vi "FPGA_Check_Pins_host.vi"() -> ()   [LabVIEW 2018]
uses:
  <vilib>/userdefined/High Color/nirio_resource_hc.ctl
  <vilib>/FPGAPlugInAG/PXI-7951R/niLvFpga_Open_PXI-7951R.vi
  <vilib>/rvi/interface/common/dynamic/niFpgaDynamicAddResources.vi
  <vilib>/FPGAPlugInAG/Dynamic/niLvFpga_Reset_Dynamic.vi
  <vilib>/FPGAPlugInAG/Dynamic/niLvFpga_Run_Dynamic.vi
  <vilib>/Utility/error.llb/Error Cluster From Error Code.vi
  <vilib>/rvi/errors/niLvFpgaAdjustHostInterfaceError.vi
  <vilib>/FPGAPlugInAG/Dynamic/niLvFpga_Close_Dynamic.vi
  <vilib>/rvi/interface/nirviOpenFPGA/nirviOpenFPGA.xnode
  FPGA Bitfiles/FPGACheckPins_FPGATarget_FPGACheckPinstar_hYVdCtpyRbw.lvbitx
  <vilib>/rvi/interface/nirviMethod/nirviMethod.xnode
  <vilib>/rvi/interface/nirviReadWriteControl/nirviReadWriteControl.xnode
  <vilib>/rvi/interface/nirviCloseFPGA/nirviCloseFPGA.xnode
  <vilib>/rvi/interface/Simulation/niFpgaSimulationCallBeginRW.vi
  NiFpgaLv.dll
panel:
  in  "Tab Control":T1(tab)
  out "output array":bool[][](array[boolean])
  out "appended array":bool[](array[boolean])
  out "Ток, А":dbl(knob) scale=0.0..1.0
  in  "FPGA slot name":T2="PXI1Slot2" caption="RIO Device"
  out "error out (4110)":errorcluster
  out "error out FPGA":errorcluster
  in  "Power Resource":refnum<k15>="PXI1Slot3"
  in  "Output enabled CH1":bool
  in  "Stop Program":bool
  in  "Write to Read":bool
  out "Read B":u32=117440511 format="%b"
  out "Read A":u32=134217727 format="%b"
  out "WRITE TOTAL":u32=38686286 format="%b"
  in  "Ток, А  2":dbl=0.9 caption="Current limit CH1" format="%#_13g"
  in  "Напряжение, В":dbl=3.0
  in  "Write to port":u16(ring)=1 items=["Manual mode", "Random", "Increment", "Chess", "NChess", "Only one", "Zero", "Chess diagonal", "NChess diagonal"]
  out "Delay A to B, нс":i16
  out "Delay B to A, нс":i16
  in  "Max тактов":i16
  in  "Write to PFI":u16(ring)=1 items=["Manual mode", "Random", "Increment", "Chess", "NChess", "Only one", "Zero", "Check one"]
  out "Delay 0.0, нс":i16
  out "Delay 0.1, нс":i16
  out "Delay 0.2, нс":i16
  out "Delay 0.3, нс":i16
  out "Delay 0.4, нс":i16
  out "Delay 0.5, нс":i16
  out "Delay 0.6, нс":i16
  out "Delay 0.7, нс":i16
  out "Delay 1.0, нс":i16
  out "Delay 1.1, нс":i16
  out "Delay 1.2, нс":i16
  out "Delay 1.3, нс":i16
  out "Delay 1.4, нс":i16
  out "Delay 1.5, нс":i16
  out "Delay 1.6, нс":i16
  out "Delay 1.7, нс":i16
  out "Delay 2.0, нс":i16
  out "Delay 2.1, нс":i16
  out "Delay 2.2, нс":i16
  out "Delay 2.3, нс":i16
  out "Delay 2.4, нс":i16
  out "Delay 2.5, нс":i16
  out "Delay 2.6, нс":i16
  out "Delay 2.7, нс":i16
  out "Delay PFI1, нс":i16
  out "Delay PFI2, нс":i16
  out "Delay PFI3, нс":i16
  in  "milliseconds to wait":u32
  out "Delay 0.0, нс":i16
  out "Delay 0.1, нс":i16
  out "Delay 0.2, нс":i16
  out "Delay 0.3, нс":i16
  out "Delay 0.4, нс":i16
  out "Delay 0.5, нс":i16
  out "Delay 0.6, нс":i16
  out "Delay 0.7, нс":i16
  out "Delay 1.0, нс":i16
  out "Delay 1.1, нс":i16
  out "Delay 1.2, нс":i16
  out "Delay 1.3, нс":i16
  out "Delay 1.4, нс":i16
  out "Delay 1.5, нс":i16
  out "Delay 1.6, нс":i16
  out "Delay 1.7, нс":i16
  out "Delay 2.0, нс":i16
  out "Delay 2.1, нс":i16
  out "Delay 2.2, нс":i16
  out "Delay 2.3, нс":i16
  out "Delay 2.4, нс":i16
  out "Delay 2.5, нс":i16
  out "Delay 2.6, нс":i16
  out "Delay 2.7, нс":i16
  out "Delay PFI1, нс":i16
  out "Delay PFI2, нс":i16
  out "Delay PFI3, нс":i16
  out "U CH0.1, В":dbl=0.000596728952024882
  out "I CH0.1, A":dbl=2.324707150327661e-06
  in  "Write to PFI 2":u8=6 format="%b"
  in  "Cycle":bool=TRUE
  in  "Write to port  2":u8=248 format="%b"
  out "Read PFI 2":i16=1
  out "Read PFI 3":i16=1
  out "Read PFI 1":i16
  out "Чтение PFI 1":i16=1
  out "Чтение PFI 2":i16=1
  out "Чтение PFI 3":i16=1
  out "Read B2":u32=255 format="%b"
  out "Read B1":u32=255 format="%b"
  out "Read B0":u32=255 format="%b"
  out "Read А2":u32=255 format="%b"
  out "Read А1":u32=255 format="%b"
  out "Read А0":u32=255 format="%b"
  # "0          1          2         3          4          5          6          7"
  # "Port 0"
  # "PFI 1"
  # "Port 1"
  # "PFI 2"
  # "Port 2"
  # "PFI 3"
  # "0 канал"
  # "1 канал"
  # "2 канал"
  # "PFI"
  # "1 канал"
  # "2 канал"
  # "PFI"
  # "0 канал"
  # "Control"
  # "Чтение портов"
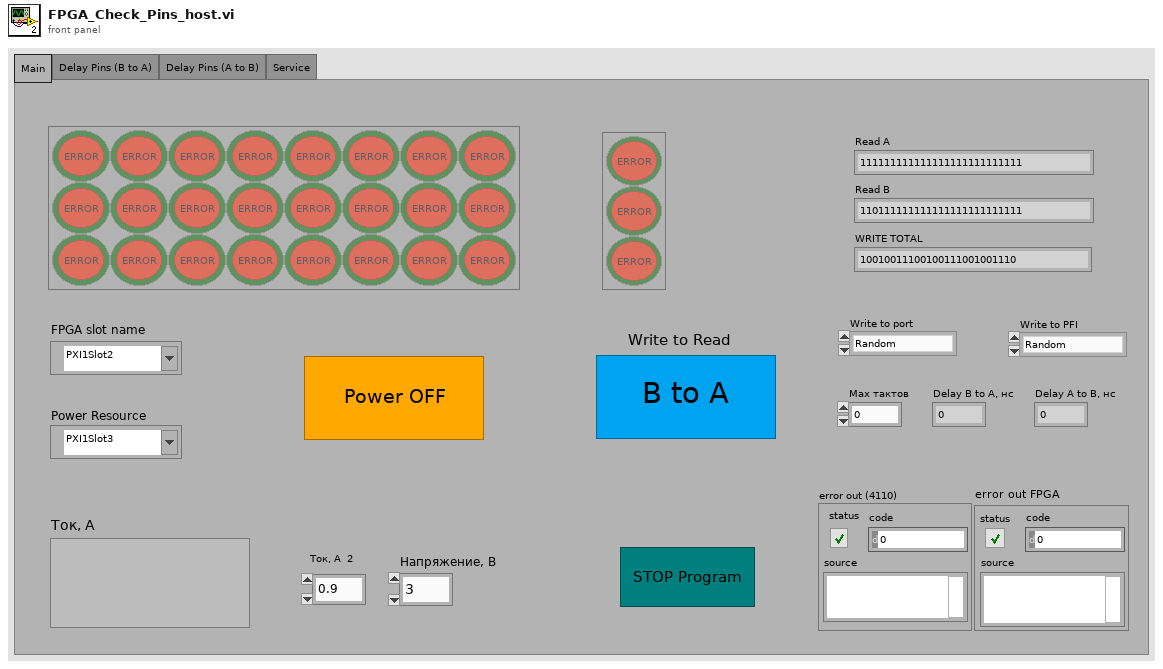
[diagram p1: front panel]
types:
  T1 = enum32{"Main", "Delay Pins (B to A)", "Delay Pins (A to B)", "Service"}
  T2 = typedef "nirio_resource_hc.ctl" = tag
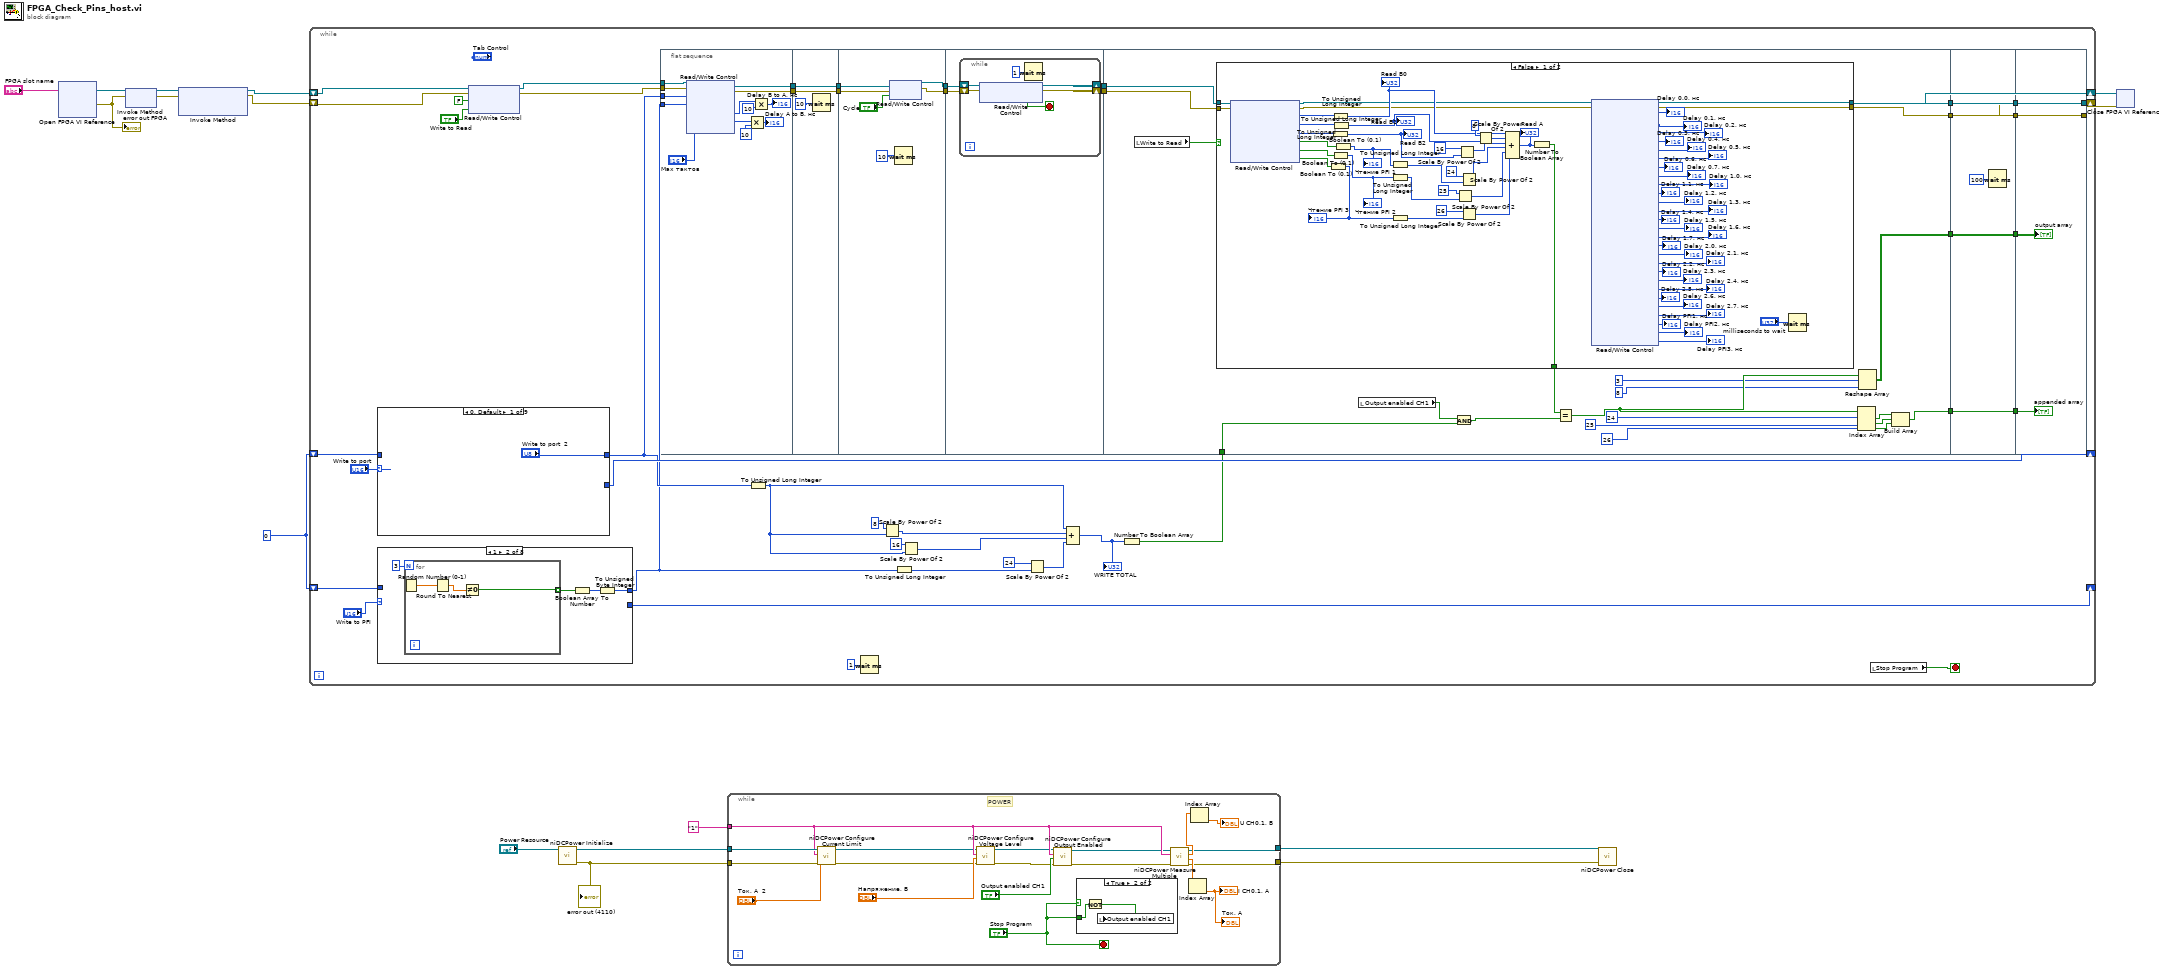
[diagram p0: block diagram]
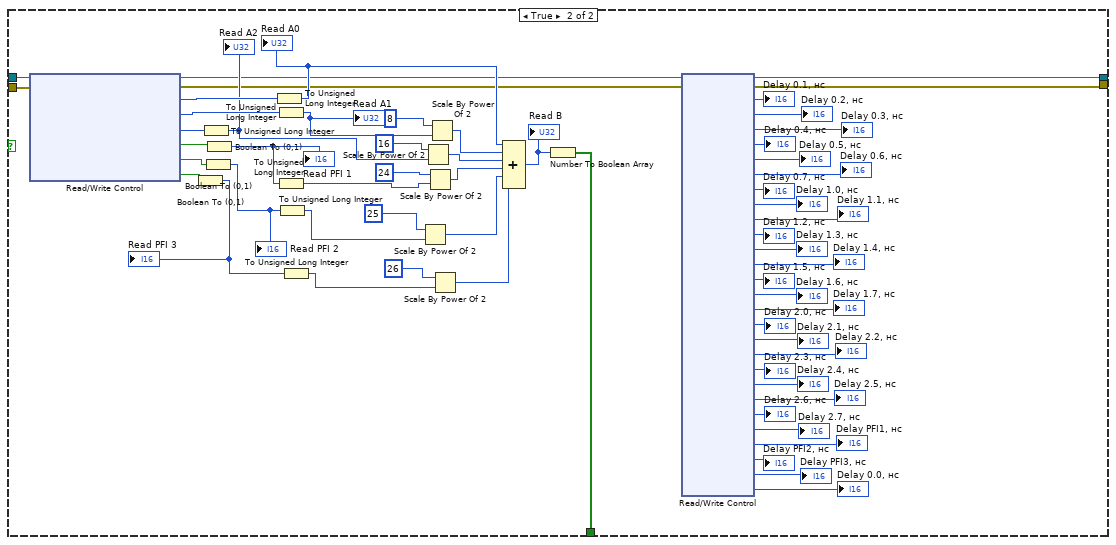
[diagram p2: hidden frame]
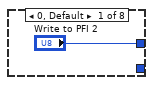
[diagram p3: hidden frame]
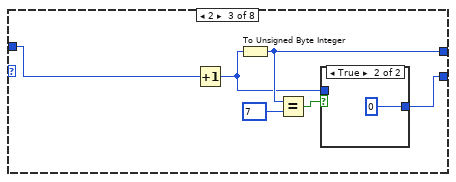
[diagram p4: hidden frame]
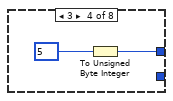
[diagram p6: hidden frame]
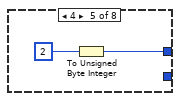
[diagram p7: hidden frame]
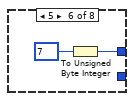
[diagram p8: hidden frame]
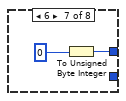
[diagram p9: hidden frame]
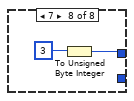
[diagram p10: hidden frame]
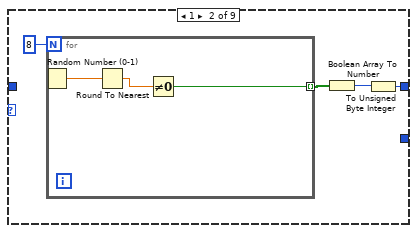
[diagram p11: hidden frame]
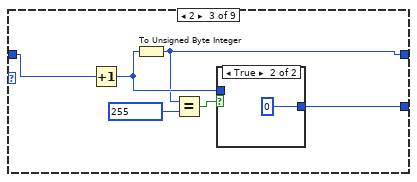
[diagram p12: hidden frame]
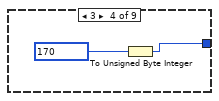
[diagram p14: hidden frame]
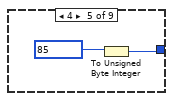
[diagram p15: hidden frame]
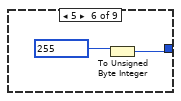
[diagram p16: hidden frame]
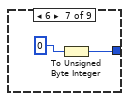
[diagram p17: hidden frame]
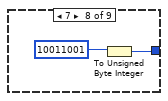
[diagram p18: hidden frame]
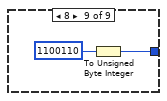
[diagram p19: hidden frame]
diagram:
  w1 = 0
  n1 = xnode "Open FPGA VI Reference"("resource name"="FPGA slot name") -> ("FPGA VI Reference Out"=w9:refnum<k20>, "error out"=w8:errorcluster)  [unwired: 1 in]
  "error out FPGA" <- w8
  n2 = xnode "Invoke Method"("FPGA VI Reference In"=w9, "error in"=w8) -> ("FPGA VI Reference Out"=w7:refnum<k20>, "error out"=w6:errorcluster)
  n3 = xnode ("Invoke Method")("FPGA VI Reference In"=w7, "error in"=w6) -> ("FPGA VI Reference Out"=w3:refnum<k20>, "error out"=w2:errorcluster)  [unwired: 1 in]
  n4 = while {
    shift-right: [w27] -> w5
    shift-left: w3 -> [w45]
    shift-right: [w26] -> w4
    shift-left: w2 -> [w44]
    shift-right: [w48] -> _
    shift-left: w1 -> [w49]
    shift-right: [w46] -> _
    shift-left: w1 -> [w47]
    stop <- w30 stop-if-true
    n5 = case shown="0, Default" "Write to port" {
      tunnel: ["Write to port  2" w270 w278 w285 w288 w290 w292 w294 w295] -> w41
      tunnel: w47 -> [_ _ w279 _ _ _ _ _ _]
      tunnel: [_ _ w277 _ _ _ _ _ _] -> w46
      frame 0, Default {
      }
      frame 1 {
        n6 = for {
          N: 8 -> [_]
          tunnel: [w274] -> w272 mode=indexing
          n7 = Random Number (0-1)() -> (number: 0 to 1=w276:dbl)
          n8 = Round To Nearest(number=w276) -> (nearest integer value=w275:dbl)
          n9 = Not Equal To 0?(x=w275) -> (x != 0?=w274:bool)
        }
        n10 = Boolean Array To Number(Boolean array=w272) -> (number=w271:u32)
        n11 = To Unsigned Byte Integer(number=w271) -> (unsigned 8bit integer=w270:u8)
      }
      frame 2 {
        n12 = Increment(x=w279) -> (x+1=w282:i32)
        n13 = To Unsigned Byte Integer(number=w282) -> (unsigned 8bit integer=w278:u8)
        n14 = Equal?(x=w278, y=u8 255) -> (x = y?=w281:bool)
        n15 = case shown="True" w281 {
          tunnel: [w283 0] -> w277
          tunnel: w282 -> [w283 _]
          frame False {
          }
          frame True {
          }
        }
      }
      frame 3 {
        n16 = To Unsigned Byte Integer(number=170) -> (unsigned 8bit integer=w285:u8)
      }
      frame 4 {
        n17 = To Unsigned Byte Integer(number=85) -> (unsigned 8bit integer=w288:u8)
      }
      frame 5 {
        n18 = To Unsigned Byte Integer(number=255) -> (unsigned 8bit integer=w290:u8)
      }
      frame 6 {
        n19 = To Unsigned Byte Integer(number=0) -> (unsigned 8bit integer=w292:u8)
      }
      frame 7 {
        n20 = To Unsigned Byte Integer(number=10011001) -> (unsigned 8bit integer=w294:u8)
      }
      frame 8 {
        n21 = To Unsigned Byte Integer(number=1100110) -> (unsigned 8bit integer=w295:u8)
      }
    }
    n22 = case shown="1" "Write to PFI" {
      tunnel: ["Write to PFI 2" w244 w254 w260 w262 w264 w266 w268] -> w38
      tunnel: w49 -> [_ _ w256 _ _ _ _ _]
      tunnel: [_ _ w252 _ _ _ _ _] -> w48
      frame 0, Default {
      }
      frame 1 {
        n23 = for {
          N: 3 -> [_]
          tunnel: [w248] -> w246 mode=indexing
          n24 = Random Number (0-1)() -> (number: 0 to 1=w250:dbl)
          n25 = Round To Nearest(number=w250) -> (nearest integer value=w249:dbl)
          n26 = Not Equal To 0?(x=w249) -> (x != 0?=w248:bool)
        }
        n27 = Boolean Array To Number(Boolean array=w246) -> (number=w245:u32)
        n28 = To Unsigned Byte Integer(number=w245) -> (unsigned 8bit integer=w244:u8)
      }
      frame 2 {
        n29 = Increment(x=w256) -> (x+1=w251:i32)
        n30 = To Unsigned Byte Integer(number=w251) -> (unsigned 8bit integer=w254:u8)
        n31 = Equal?(x=w254, y=u8 7) -> (x = y?=w253:bool)
        n32 = case shown="True" w253 {
          tunnel: [w257 0] -> w252
          tunnel: w251 -> [w257 _]
          frame False {
          }
          frame True {
          }
        }
      }
      frame 3 {
        n33 = To Unsigned Byte Integer(number=5) -> (unsigned 8bit integer=w260:u8)
      }
      frame 4 {
        n34 = To Unsigned Byte Integer(number=2) -> (unsigned 8bit integer=w262:u8)
      }
      frame 5 {
        n35 = To Unsigned Byte Integer(number=7) -> (unsigned 8bit integer=w264:u8)
      }
      frame 6 {
        n36 = To Unsigned Byte Integer(number=0) -> (unsigned 8bit integer=w266:u8)
      }
      frame 7 {
        n37 = To Unsigned Byte Integer(number=3) -> (unsigned 8bit integer=w268:u8)
      }
    }
    n38 = xnode "Read/Write Control"("FPGA VI Reference In"=w45, "error in"=w44, "Cycle"=FALSE, "A to B/B to A"="Write to Read") -> ("FPGA VI Reference Out"=w43:refnum<k20>, "error out"=w42:errorcluster)
    n39 = flat-sequence {
      tunnel: w43 -> [w71]
      tunnel: w42 -> [w70]
      tunnel: w41 -> [w69]
      tunnel: w38 -> [w68]
      tunnel: [w73] -> w37
      tunnel: [w72] -> w36
      tunnel: w37 -> [w76]
      tunnel: w36 -> [w75]
      tunnel: [w76] -> w35
      tunnel: [w75] -> w34
      tunnel: w35 -> [w82]
      tunnel: w34 -> [w81]
      tunnel: [w80] -> w33
      tunnel: [w79] -> w32
      tunnel: w33 -> [w84]
      tunnel: w32 -> [w83]
      tunnel: [w86] -> w29
      tunnel: [w85] -> w28
      tunnel: w29 -> [w111]
      tunnel: w28 -> [w110]
      tunnel: w25 -> [w107]
      tunnel: [w109] -> w24
      tunnel: [w108] -> w23
      tunnel: [w94] -> w19
      tunnel: [w93] -> w17
      tunnel: w24 -> [w238]
      tunnel: w23 -> [w237]
      tunnel: [w238] -> w22
      tunnel: [w237] -> w21
      tunnel: [w236] -> w20
      tunnel: w19 -> [w236]
      tunnel: [w235] -> w18
      tunnel: w17 -> [w235]
      tunnel: [w241] -> w26
      tunnel: [w242] -> w27
      tunnel: w22 -> [w242]
      tunnel: w21 -> [w241]
      tunnel: w20 -> [w240]
      tunnel: w18 -> [w239]
      frame #0 {
        n40 = xnode "Read/Write Control"("FPGA VI Reference In"=w71, "error in"=w70, "Write to"=w69, "Write to PFI"=w68, "Counter"="Max тактов") -> ("FPGA VI Reference Out"=w73:refnum<k20>, "error out"=w72:errorcluster, "Delay B to A"=w65:i16, "Delay A to B"=w61:i16)
        n41 = Multiply(x=w61, y=i16 10) -> (x*y=→"Delay A to B, нс":i16)
        n42 = Multiply(x=w65, y=i16 10) -> (x*y=→"Delay B to A, нс":i16)
      }
      frame #1 {
        n43 = Wait (ms)(milliseconds to wait=u32 10) -> ()  [unwired: 1 out]
      }
      frame #2 {
        n44 = xnode "Read/Write Control"("FPGA VI Reference In"=w82, "error in"=w81, "Cycle"="Cycle") -> ("FPGA VI Reference Out"=w80:refnum<k20>, "error out"=w79:errorcluster)
        n45 = Wait (ms)(milliseconds to wait=u32 10) -> ()  [unwired: 1 out]
      }
      frame #3 {
        n46 = while {
          shift-right: [w92] -> w86
          shift-left: w84 -> [w90]
          shift-right: [w91] -> w85
          shift-left: w83 -> [w89]
          stop <- w87 stop-if-true
          n47 = xnode "Read/Write Control"("FPGA VI Reference In"=w90, "error in"=w89) -> ("FPGA VI Reference Out"=w92:refnum<k20>, "error out"=w91:errorcluster, "Operation compl"=w87:bool)
          n48 = Wait (ms)(milliseconds to wait=u32 1) -> ()  [unwired: 1 out]
        }
      }
      frame #4 {
        n49 = local read "Write to Read"() -> (w112:bool)
        n50 = case shown="False" w112 {
          tunnel: [w142 w203] -> w109
          tunnel: [w141 w202] -> w108
          tunnel: [w163 w229] -> w104
          tunnel: w111 -> [w146 w206]
          tunnel: w110 -> [w145 w205]
          frame False {
            n51 = xnode "Read/Write Control"("FPGA VI Reference In"=w146, "error in"=w145) -> ("FPGA VI Reference Out"=w144:refnum<k20>, "error out"=w143:errorcluster, "Read Port 0 A"=w169:u8, "Read Port 1 A"=w168:u8, "Read Port 2 A"=w167:u8, "DDCA_PFI1_Read 3"=w159:bool, "DDCA_PFI2_Read 3"=w157:bool, "DDCA_PFI3_Read 3"=w158:bool)
            n52 = Boolean To (0,1)(Boolean=w158) -> (0, 1=w150:i16)
            "Чтение PFI 3" <- w150
            n53 = To Unsigned Long Integer(number=w167) -> (unsigned 32bit integer=w166:u32)
            "Read B2" <- w166
            n54 = To Unsigned Long Integer(number=w169) -> (unsigned 32bit integer=w164:u32)
            "Read B0" <- w164
            n55 = Boolean To (0,1)(Boolean=w157) -> (0, 1=w151:i16)
            "Чтение PFI 2" <- w151
            n56 = To Unsigned Long Integer(number=w168) -> (unsigned 32bit integer=w165:u32)
            "Read B1" <- w165
            n57 = Boolean To (0,1)(Boolean=w159) -> (0, 1=w152:i16)
            "Чтение PFI 1" <- w152
            n58 = To Unsigned Long Integer(number=w152) -> (unsigned 32bit integer=w147:u32)
            n59 = To Unsigned Long Integer(number=w151) -> (unsigned 32bit integer=w148:u32)
            n60 = To Unsigned Long Integer(number=w150) -> (unsigned 32bit integer=w149:u32)
            n61 = Scale By Power Of 2(n=i16 25, x=w148) -> (x*2^n=w156:u32)
            n62 = Scale By Power Of 2(n=i16 16, x=w166) -> (x*2^n=w162:u32)
            n63 = Scale By Power Of 2(n=i16 24, x=w147) -> (x*2^n=w161:u32)
            n64 = Scale By Power Of 2(n=i16 26, x=w149) -> (x*2^n=w155:u32)
            n65 = Scale By Power Of 2(n=i16 8, x=w165) -> (x*2^n=w172:u32)
            n66 = Compound Arithmetic op=unknown(w164, w172, w162, w161, w156, w155) -> (w173:u32)
            "Read A" <- w173
            n67 = Number To Boolean Array(number=w173) -> (Boolean array=w163:bool[])
            n68 = xnode "Read/Write Control"("FPGA VI Reference In"=w144, "error in"=w143) -> ("FPGA VI Reference Out"=w142:refnum<k20>, "error out"=w141:errorcluster, "Delay 0.0 (B to A)"=→"Delay 0.0, нс":i16, "Delay 0.1 (B to A)"=→"Delay 0.1, нс":i16, "Delay 0.2 (B to A)"=→"Delay 0.2, нс":i16, "Delay 0.3 (B to A)"=→"Delay 0.3, нс":i16, "Delay 0.4 (B to A)"=→"Delay 0.4, нс":i16, "Delay 0.5 (B to A)"=→"Delay 0.5, нс":i16, "Delay 0.6 (B to A)"=→"Delay 0.6, нс":i16, "Delay 0.7 (B to A)"=→"Delay 0.7, нс":i16, "Delay 1.0 (B to A)"=→"Delay 1.0, нс":i16, "Delay 1.1 (B to A)"=→"Delay 1.1, нс":i16, "Delay 1.2 (B to A)"=→"Delay 1.2, нс":i16, "Delay 1.3 (B to A)"=→"Delay 1.3, нс":i16, "Delay 1.4 (B to A)"=→"Delay 1.4, нс":i16, "Delay 1.5 (B to A)"=→"Delay 1.5, нс":i16, "Delay 1.6 (B to A)"=→"Delay 1.6, нс":i16, "Delay 1.7 (B to A)"=→"Delay 1.7, нс":i16, "Delay 2.0 (B to A)"=→"Delay 2.0, нс":i16, "Delay 2.1 (B to A)"=→"Delay 2.1, нс":i16, "Delay 2.2 (B to A)"=→"Delay 2.2, нс":i16, "Delay 2.3 (B to A)"=→"Delay 2.3, нс":i16, "Delay 2.4 (B to A)"=→"Delay 2.4, нс":i16, "Delay 2.5 (B to A)"=→"Delay 2.5, нс":i16, "Delay 2.6 (B to A)"=→"Delay 2.6, нс":i16, "Delay 2.7 (B to A)"=→"Delay 2.7, нс":i16, "Delay PFI1 (B to A)"=→"Delay PFI1, нс":i16, "Delay PFI2 (B to A)"=→"Delay PFI2, нс":i16, "Delay PFI3 (B to A)"=→"Delay PFI3, нс":i16)
            n69 = Wait (ms)(milliseconds to wait="milliseconds to wait") -> ()  [unwired: 1 out]
          }
          frame True {
            n70 = xnode ("Read/Write Control")("FPGA VI Reference In"=w206, "error in"=w205) -> ("FPGA VI Reference Out"=w204:refnum<k20>, "error out"=w201:errorcluster, "Read Port 0 B"=w228:u8, "Read Port 1 B"=w225:u8, "Read Port 2 B"=w224:u8, "DDCB_PFI1_Read (A to B)"=w218:bool, "DDCB_PFI2_Read (A to B)"=w219:bool, "DDCB_PFI3_Read (A to B)"=w220:bool)
            n71 = Boolean To (0,1)(Boolean=w220) -> (0, 1=w212:i16)
            "Read PFI 3" <- w212
            n72 = To Unsigned Long Integer(number=w224) -> (unsigned 32bit integer=w223:u32)
            "Read А2" <- w223
            n73 = Boolean To (0,1)(Boolean=w219) -> (0, 1=w209:i16)
            "Read PFI 2" <- w209
            n74 = Boolean To (0,1)(Boolean=w218) -> (0, 1=w208:i16)
            "Read PFI 1" <- w208
            n75 = To Unsigned Long Integer(number=w228) -> (unsigned 32bit integer=w227:u32)
            "Read А0" <- w227
            n76 = To Unsigned Long Integer(number=w225) -> (unsigned 32bit integer=w226:u32)
            "Read А1" <- w226
            n77 = To Unsigned Long Integer(number=w208) -> (unsigned 32bit integer=w207:u32)
            n78 = To Unsigned Long Integer(number=w209) -> (unsigned 32bit integer=w210:u32)
            n79 = To Unsigned Long Integer(number=w212) -> (unsigned 32bit integer=w211:u32)
            n80 = Scale By Power Of 2(n=i16 25, x=w210) -> (x*2^n=w216:u32)
            n81 = Scale By Power Of 2(n=i16 16, x=w223) -> (x*2^n=w232:u32)
            n82 = Scale By Power Of 2(n=24, x=w207) -> (x*2^n=w217:u32)
            n83 = Scale By Power Of 2(n=i16 8, x=w226) -> (x*2^n=w233:u32)
            n84 = Scale By Power Of 2(n=i16 26, x=w211) -> (x*2^n=w215:u32)
            n85 = Compound Arithmetic op=unknown(w227, w233, w232, w217, w216, w215) -> (w230:u32)
            "Read B" <- w230
            n86 = Number To Boolean Array(number=w230) -> (Boolean array=w229:bool[])
            n87 = xnode "Read/Write Control"("FPGA VI Reference In"=w204, "error in"=w201) -> ("FPGA VI Reference Out"=w203:refnum<k20>, "error out"=w202:errorcluster, "Delay 0.1"=→"Delay 0.1, нс":i16, "Delay 0.2"=→"Delay 0.2, нс":i16, "Delay 0.3"=→"Delay 0.3, нс":i16, "Delay 0.4"=→"Delay 0.4, нс":i16, "Delay 0.5"=→"Delay 0.5, нс":i16, "Delay 0.6"=→"Delay 0.6, нс":i16, "Delay 0.7"=→"Delay 0.7, нс":i16, "Delay 1.0"=→"Delay 1.0, нс":i16, "Delay 1.1"=→"Delay 1.1, нс":i16, "Delay 1.2"=→"Delay 1.2, нс":i16, "Delay 1.3"=→"Delay 1.3, нс":i16, "Delay 1.4"=→"Delay 1.4, нс":i16, "Delay 1.5"=→"Delay 1.5, нс":i16, "Delay 1.6"=→"Delay 1.6, нс":i16, "Delay 1.7"=→"Delay 1.7, нс":i16, "Delay 2.0"=→"Delay 2.0, нс":i16, "Delay 2.1"=→"Delay 2.1, нс":i16, "Delay 2.2"=→"Delay 2.2, нс":i16, "Delay 2.3"=→"Delay 2.3, нс":i16, "Delay 2.4"=→"Delay 2.4, нс":i16, "Delay 2.5"=→"Delay 2.5, нс":i16, "Delay 2.6"=→"Delay 2.6, нс":i16, "Delay 2.7"=→"Delay 2.7, нс":i16, "Delay PFI1"=→"Delay PFI1, нс":i16, "Delay PFI2"=→"Delay PFI2, нс":i16, "Delay PFI3"=→"Delay PFI3, нс":i16, "Delay 0.0"=→"Delay 0.0, нс":i16)
          }
        }
        n88 = local read "Output enabled CH1"() -> (w106:bool)
        n89 = And(x=w106, y=w107) -> (x .and. y?=w105:bool[])
        n90 = Equal?(x=w104, y=w105) -> (x = y?=w100:bool[])
        n91 = Index Array(array=w100, index #1=24 ("index"), index #2=25 ("index"), index #3=26 ("index")) -> (element #1=w101:bool, element #2=w102:bool, element #3=w103:bool)
        n92 = Reshape Array(w100, 3 ("dimension size"), 8 ("dimension size")) -> (w94:bool[][])
        n93 = Build Array(w101, w102, w103) -> (w93:bool[])
      }
      frame #5 {
        n94 = Wait (ms)(milliseconds to wait=u32 100) -> ()  [unwired: 1 out]
      }
      frame #6 {
        "output array" <- w240
        "appended array" <- w239
      }
    }
    n95 = To Unsigned Long Integer(number=w41) -> (unsigned 32bit integer=w55:u32)
    n96 = Wait (ms)(milliseconds to wait=u32 1) -> ()  [unwired: 1 out]
    n97 = Scale By Power Of 2(n=i16 8, x=w55) -> (x*2^n=w59:u32)
    n98 = To Unsigned Long Integer(number=w38) -> (unsigned 32bit integer=w54:u32)
    n99 = Scale By Power Of 2(n=i16 16, x=w55) -> (x*2^n=w60:u32)
    n100 = Scale By Power Of 2(n=i16 24, x=w54) -> (x*2^n=w52:u32)
    n101 = Compound Arithmetic op=ADD(w55, w59, w60, w52) -> (w58:u32)
    "WRITE TOTAL" <- w58
    n102 = Number To Boolean Array(number=w58) -> (Boolean array=w25:bool[])
    n103 = local read "Stop Program"() -> (w30:bool)
  }
  n104 = call <instrlib>:"niDCPower Initialize.vi"("resource name"="Power Resource") -> ("error out"=w15:errorcluster, "instrument handle out"=w14:refnum<k15>)  [unwired: 3 in, 6 out]
  "error out (4110)" <- w15
  n105 = while {
    tunnel: [w303] -> w12
    tunnel: [w302] -> w13
    tunnel: "1" ("Channel name") -> [w308]
    tunnel: w15 -> [w309]
    tunnel: w14 -> [w310]
    stop <- "Stop Program" stop-if-true
    # "POWER"
    n106 = call <instrlib>:"niDCPower Configure Current Limit.vi"("error in (no error)"=w309, "current limit"="Ток, А  2", "channel name"=w308, "instrument handle"=w310) -> ("error out"=w307:errorcluster, "instrument handle out"=w306:refnum<k15>)  [unwired: 6 in]
    n107 = call <instrlib>:"niDCPower Configure Voltage Level.vi"("error in (no error)"=w307, "voltage level"="Напряжение, В", "channel name"=w308, "instrument handle"=w306) -> ("error out"=w304:errorcluster, "instrument handle out"=w305:refnum<k15>)  [unwired: 6 in]
    n108 = call <instrlib>:"niDCPower Configure Output Enabled.vi"("error in (no error)"=w304, "output enabled"="Output enabled CH1", "channel name"=w308, "instrument handle"=w305) -> ("error out"=w300:errorcluster, "instrument handle out"=w301:refnum<k15>)  [unwired: 6 in]
    n109 = case shown="True" "Stop Program" {
      tunnel: "Stop Program" -> [_ w317]
      frame False {
      }
      frame True {
        n110 = Not(x=w317) -> (.not. x?=w316:bool)
        n111 = local write "Output enabled CH1"(w316) -> ()
      }
    }
    n112 = call <instrlib>:"niDCPower Measure Multiple.vi"("error in (no error)"=w300, "channel name"=w308, "instrument handle"=w301) -> ("error out"=w303:errorcluster, "current measurements"=w314:dbl[], "voltage measurements"=w312:dbl[], "instrument handle out"=w302:refnum<k15>)  [unwired: 5 in]
    n113 = Index Array(array=w314) -> (element=→"I CH0.1, A" →"Ток, А":dbl)  [unwired: 1 in]
    n114 = Index Array(array=w312) -> (element=→"U CH0.1, В":dbl)  [unwired: 1 in]
  }
  n115 = call <instrlib>:"niDCPower Close.vi"("error in (no error)"=w12, "instrument handle"=w13) -> ()  [unwired: 9 in, 1 out]
  n116 = xnode "Close FPGA VI Reference"("FPGA VI Reference In"=w5, "error in"=w4) -> ()  [unwired: 1 out]
